vi "Quarternion SLERP.vi"(8 "error in (no error)":errorcluster, 9 "Factor":dbl, 10 "To":T1, 11 "From":T1) -> (0 "error out":errorcluster, 3 "SLERP Result":T1)   [LabVIEW 2020, in "ar.lvlib"]
doc: "Interpolate between two Quaternions."
uses:
  ar.lvlib
  Quaternion.ctl
  common/common.lvlib
  common/bin/gartoolkit_ar_32-1.dll
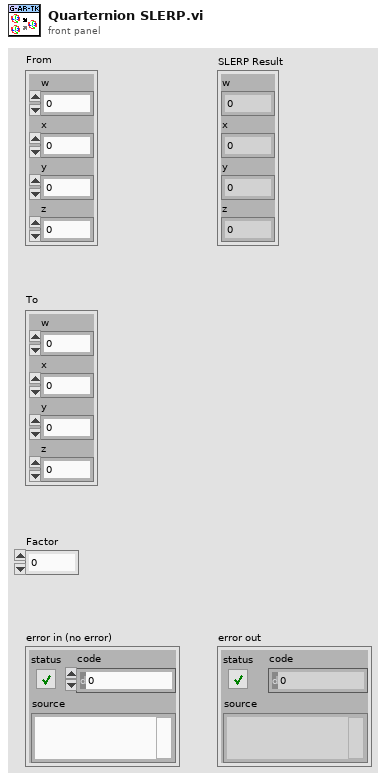
[diagram p1: front panel]
types:
  T1 = typedef "ar.lvlib/Quaternion.ctl" = cluster{"w":dbl, "x":dbl, "y":dbl, "z":dbl}
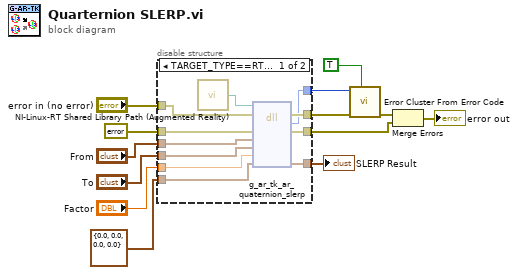
[diagram p0: block diagram]
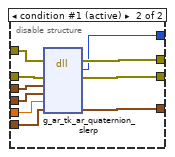
[diagram p2: hidden frame]
diagram:
  n1 = disable-structure shown="TARGET_TYPE==RT&&OS==Linux" {
    disable-tunnel: "error in (no error)" -> [w24 w34]
    disable-tunnel: errorcluster {"status"=FALSE, "code"=0, "source"=""} ("error constant") -> [w23 w33]
    disable-tunnel: "From" -> [w22 w32]
    disable-tunnel: "To" -> [w21 w31]
    disable-tunnel: "Factor" -> [w20 w30]
    disable-tunnel: T1 {"w"=0.0, "x"=0.0, "y"=0.0, "z"=0.0} ("Quaternion") -> [w19 w29]
    disable-tunnel: [w18 w28] -> w5
    disable-tunnel: [w17 w27] -> w4
    disable-tunnel: [w16 w26] -> w3
    disable-tunnel: [w15 w25] -> w2
    frame condition #0 {
      n2 = call "NI-Linux-RT Shared Library Path (Augmented Reality).vi"() -> ("Path"=w14:path)
      n3 = dll-call lib="?" fn="g_ar_tk_ar_quaternion_slerp" ("g_ar_toolkit.*.*:g_ar_tk_image_copy")(path in=w14, error in=w24, "error_cluster"=w23, "from"=w22, "to"=w21, "factor"=w20, "result"=w19) -> (error out=w18:errorcluster, w17:i32, "error_cluster"=w16:errorcluster, "result"=w15:T1)  [unwired: 4 in, 1 out]
    }
    frame condition #1 (active) {
      n4 = dll-call lib="C:/serenial/lib/g-augmented-reality-toolkit/LabVIEW/common/bin/gartoolkit_ar_*-1.*" fn="g_ar_tk_ar_quaternion_slerp" ("g_ar_toolkit.*.*:g_ar_tk_image_copy")(error in=w34, "error_cluster"=w33, "from"=w32, "to"=w31, "factor"=w30, "result"=w29) -> (error out=w28:errorcluster, w27:i32, "error_cluster"=w26:errorcluster, "result"=w25:T1)  [unwired: 5 in, 1 out]
    }
  }
  "SLERP Result" <- w2
  n5 = call <vilib>:"Error Cluster From Error Code.vi"("show call chain? (False)"=TRUE, "error in (no error)"=w5, "error code (0)"=w4) -> ("error out"=w13:errorcluster)  [unwired: 6 in]
  n6 = Merge Errors(w13, w3) -> (→"error out":errorcluster)
